vi "GetDataReference.vi"(0 "Core In":refnum<class "Core.lvclass">, 11 "Error In":errorcluster) -> (4 "Core Out":refnum<class "Core.lvclass">, 8 "Data Reference":T1, 15 "Error Out":errorcluster)   [LabVIEW 2020, in "Core.lvlib" / "Core.lvclass"]
uses:
  Core.lvclass
  DataReference.ctl
  Core.lvclass/Core.ctl
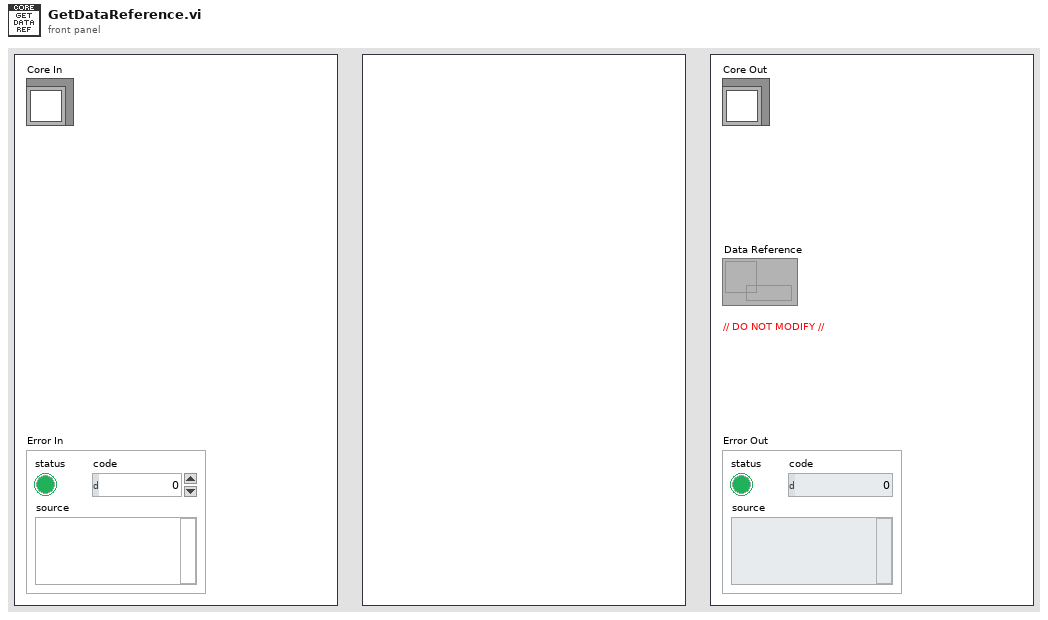
[diagram p1: front panel]
types:
  T1 = typedef "Core.lvlib/Core.lvclass/DataReference.ctl" = refnum<data-value>
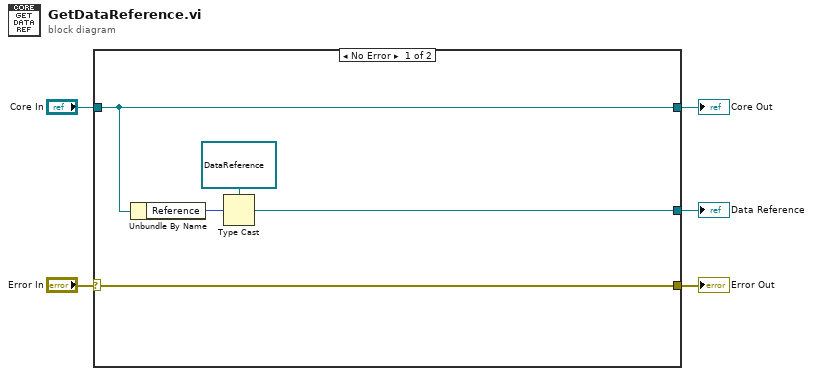
[diagram p0: block diagram]
diagram:
  n1 = case shown="No Error" "Error In" {
    selector: "Error In" -> [w10 w11]
    tunnel: [w10 w11] -> w4
    tunnel: "Core In" -> [w9 w12]
    tunnel: [w9 w12] -> w2
    tunnel: [w6 _] -> w1
    frame No Error {
      n2 = Unbundle By Name(w9) -> ("Reference"=w7:u64)
      n3 = Type Cast(type=T1 refnum ("Data Reference"), x=w7) -> (*(type *) &x=w6:T1)
    }
    frame Error {
    }
  }
  "Core Out" <- w2
  "Error Out" <- w4
  "Data Reference" <- w1
